vi "Driveshift.vi"(7 "GO BUTTON":bool, 10 "Shift down override":bool, 11 "Shift up override":bool) -> ()   [LabVIEW 2013]
uses:
  <vilib>/Rock Robotics/WPI/Solenoid/WPI_SolenoidValue.ctl
  Robot Global Data.vi
  <vilib>/Rock Robotics/WPI/Solenoid/WPI_SolenoidSetEnum.vi
panel:
  in  "Shift down":dbl=300.0
  in  "Shift up":dbl=500.0
  out "Solenoid Value":T1
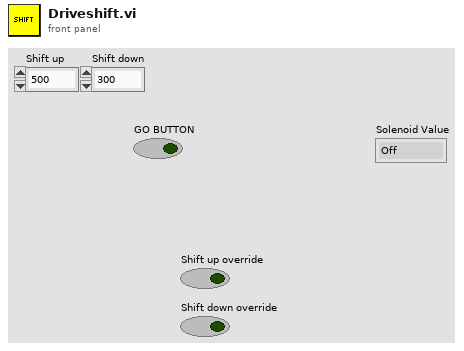
[diagram p1: front panel]
types:
  T1 = typedef "WPI_SolenoidValue.ctl" = enum16{"Off", "On", "Forward", "Reverse"}
  T2 = typedef "WPI_EncoderDevRef.ctl" = cluster{"DevStatus":errorcluster, "EncoderIndex":T3, "CounterIndex":T4, "DistancePerCount":dbl, "Decoding Type":T5}
  T3 = typedef "FPGA_EncoderIdx.ctl" = enum8{"Enc 0", "Enc 1", "Enc 2", "Enc 3", "Invalid"}
  T4 = typedef "FPGA_CounterCtrSystemIndex.ctl" = enum8{"Ctr 0", "Ctr 1", "Ctr 2", "Ctr 3", "Ctr 4", "Ctr 5", "Ctr 6", "Ctr 7", "Invalid"}
  T5 = typedef "WPI_EncoderType.ctl" = enum16{"1x", "2x", "4x"}
  T6 = typedef "WPI_SolenoidDevRef.ctl" = cluster{"DevStatus":errorcluster, "Solenoid Module":T7, "Forward Solenoid Channel":T8, "Reverse Solenoid Channel":T8}
  T7 = typedef "FPGA_TypedefSolenoidModule.ctl" = enum16{"Solenoid Module 1", "Solenoid Module 2"}
  T8 = typedef "WPI_SolenoidChannel.ctl" = enum8{"Solenoid 1", "Solenoid 2", "Solenoid 3", "Solenoid 4", "Solenoid 5", "Solenoid 6", "Solenoid 7", "Solenoid 8", "Invalid"}
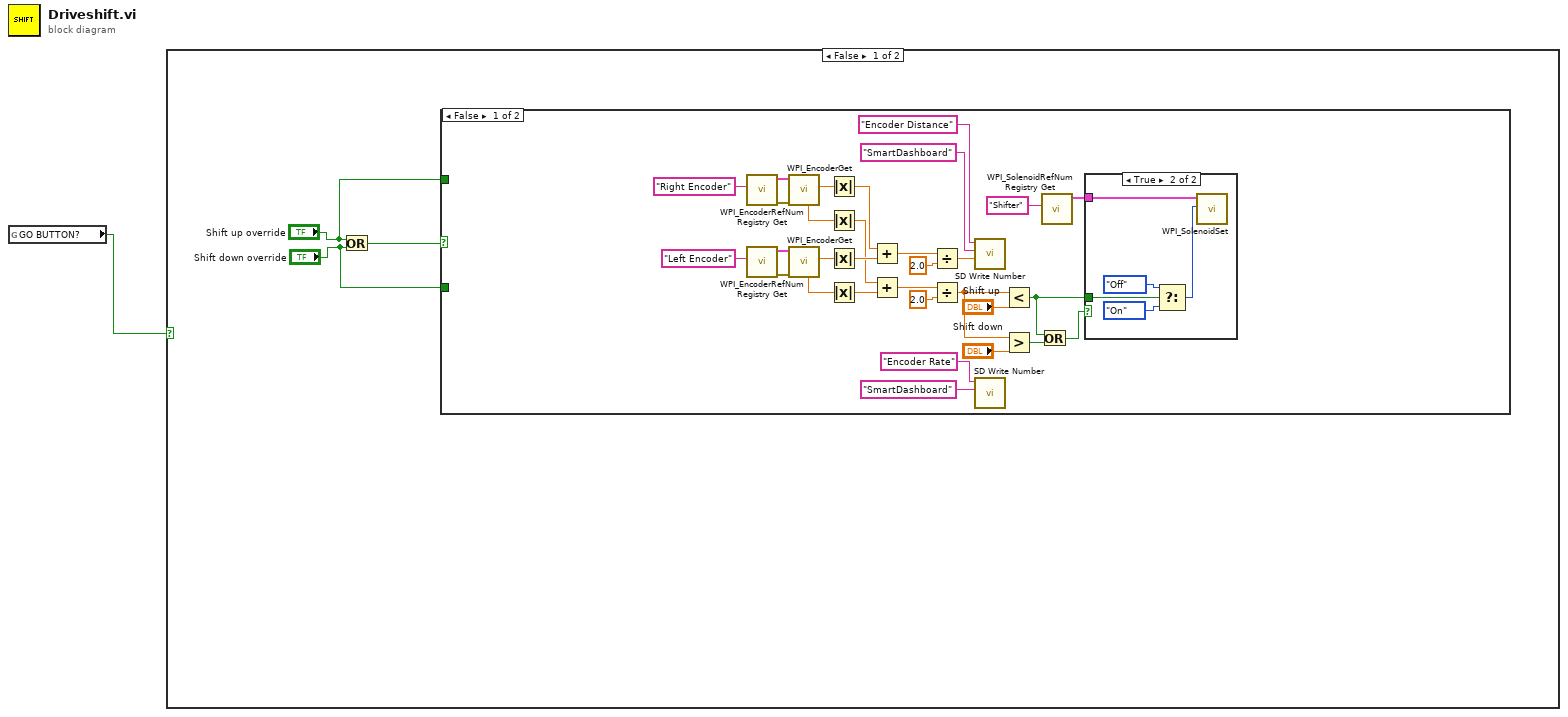
[diagram p0: block diagram]
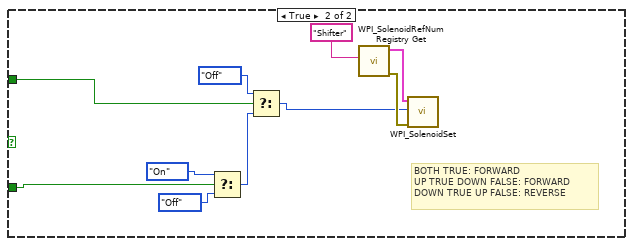
[diagram p3: hidden frame]
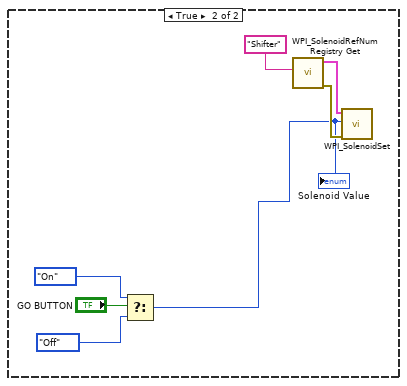
[diagram p4: hidden frame]
diagram:
  n1 = global read "Robot Global Data.vi" "GO BUTTON?"() -> (w1:bool)
  n2 = case shown="False" w1 {
    frame False {
      n3 = Or(x="Shift up override", y="Shift down override") -> (x .or. y?=w4:bool)
      n4 = case shown="False" w4 {
        tunnel: "Shift up override" -> [_ w50]
        tunnel: "Shift down override" -> [_ w48]
        frame False {
          n5 = call <vilib>:"WPI_EncoderRefNum Registry Get.vi"("refnum name"="Right Encoder") -> ("error out"=w13:errorcluster, "EncoderDevRef"=w12:T2)  [unwired: 9 in]
          n6 = call <vilib>:"WPI_EncoderRefNum Registry Get.vi"("refnum name"="Left Encoder") -> ("error out"=w10:errorcluster, "EncoderDevRef"=w11:T2)  [unwired: 9 in]
          n7 = call <vilib>:"WPI_EncoderGet.vi"("error in (no error)"=w13, "EncoderDevRef"=w12) -> ("Distance"=w21:dbl, "Rate"=w6:dbl)  [unwired: 4 in, 4 out]
          n8 = call <vilib>:"WPI_EncoderGet.vi"("error in (no error)"=w10, "EncoderDevRef"=w11) -> ("Distance"=w22:dbl, "Rate"=w5:dbl)  [unwired: 4 in, 4 out]
          n9 = Absolute Value(x=w21) -> (abs(x)=w26:dbl)
          n10 = Absolute Value(x=w6) -> (abs(x)=w23:dbl)
          n11 = Absolute Value(x=w22) -> (abs(x)=w25:dbl)
          n12 = Absolute Value(x=w5) -> (abs(x)=w24:dbl)
          n13 = Add(x=w26, y=w25) -> (x+y=w19:dbl)
          n14 = Add(x=w23, y=w24) -> (x+y=w8:dbl)
          n15 = Divide(x=w19, y=2.0) -> (x/y=w27:dbl)
          n16 = Divide(x=w8, y=2.0) -> (x/y=w28:dbl)
          n17 = call <vilib>:"SD Write Number.vi"("Numeric"=w27, "Table Prefix"="SmartDashboard", "Name"="Encoder Distance") -> ()  [unwired: 7 in, 2 out]
          n18 = call <vilib>:"SD Write Number.vi"("Table Prefix"="SmartDashboard", "Name"="Encoder Rate") -> ()  [unwired: 8 in, 2 out]
          n19 = Less?(x=w28, y="Shift up") -> (x < y?=w32:bool)
          n20 = Greater?(x=w28, y="Shift down") -> (0:w31:bool)
          n21 = Or(x=w32, y=w31) -> (x .or. y?=w33:bool)
          n22 = call <vilib>:"WPI_SolenoidRefNum Registry Get.vi"("refnum name"="Shifter") -> ("SolenoidDevRef"=w30:T6)  [unwired: 9 in, 1 out]
          n23 = case shown="True" w33 {
            tunnel: w32 -> [_ w40]
            tunnel: w30 -> [_ w36]
            frame False {
            }
            frame True {
              n24 = Select(t=WPI_SolenoidValue."Off" ("Value"), s=w40, f=WPI_SolenoidValue."On" ("Value")) -> (s? t:f=w38:T1)
              n25 = call-poly <vilib>:"WPI_SolenoidSet.vi"("Value"=w38, "SolenoidDevRef"=w36) -> ()  [unwired: 8 in, 2 out]
            }
          }
        }
        frame True {
          # "BOTH TRUE: FORWARD \nUP TRUE DOWN FALSE: FORWARD\nDOWN TRUE UP FALSE: REVERSE"
          n26 = Select(t=WPI_SolenoidValue."On" ("f"), s=w48, f=WPI_SolenoidValue."Off") -> (s? t:f=w45:T1)
          n27 = Select(t=WPI_SolenoidValue."Off" ("Value"), s=w50, f=w45) -> (s? t:f=w41:T1)
          n28 = call <vilib>:"WPI_SolenoidRefNum Registry Get.vi"("refnum name"="Shifter") -> ("error out"=w42:errorcluster, "SolenoidDevRef"=w43:T6)  [unwired: 9 in]
          n29 = call-poly <vilib>:"WPI_SolenoidSet.vi"("error in (no error)"=w42, "Value"=w41, "SolenoidDevRef"=w43) -> ()  [unwired: 7 in, 2 out]
        }
      }
    }
    frame True {
      n30 = Select(t=WPI_SolenoidValue."On" ("f"), s="GO BUTTON", f=WPI_SolenoidValue."Off") -> (s? t:f=w51:T1)
      "Solenoid Value" <- w51
      n31 = call <vilib>:"WPI_SolenoidRefNum Registry Get.vi"("refnum name"="Shifter") -> ("error out"=w52:errorcluster, "SolenoidDevRef"=w53:T6)  [unwired: 9 in]
      n32 = call-poly <vilib>:"WPI_SolenoidSet.vi"("error in (no error)"=w52, "Value"=w51, "SolenoidDevRef"=w53) -> ()  [unwired: 7 in, 2 out]
    }
  }
